vi "GetControlUID.vi"(6 "error in":errorcluster, 9 "Local in":refnum<class "Local.lvclass">) -> (0 "error out":errorcluster, 3 "Local out":refnum<class "Local.lvclass">, 4 "UID":i32)   [LabVIEW 2014, in "Local.lvclass"]
uses:
  Local.lvclass
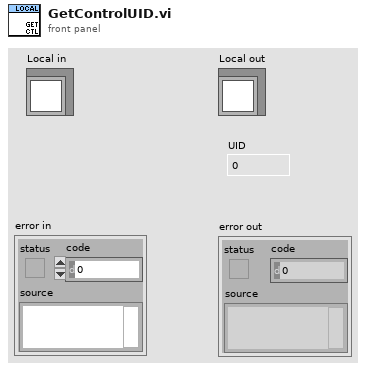
[diagram p1: front panel]
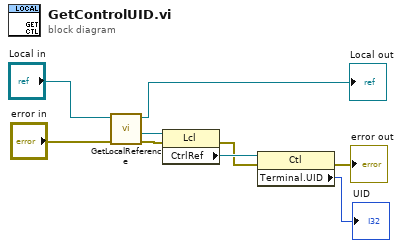
[diagram p0: block diagram]
diagram:
  n1 = call "GetLocalReference.vi"("error in"="error in", "Local in"="Local in") -> ("error out"=w5:errorcluster, "reference out"=w6:refnum<vi>, "Local out"=→"Local out":refnum<class "Local.lvclass">)  [unwired: 7 in]
  n2 = property class="Lcl"(reference=w6, error in=w5) -> (error out=w3:errorcluster, "CtrlRef"=w4:refnum<vi>)  [unwired: 1 out]
  n3 = property class="Ctl"(reference=w4, error in=w3) -> (error out=→"error out":errorcluster, "Terminal.UID"=→"UID":i32)  [unwired: 1 out]
